vi "I16ArrayToStr(cast).vi"(1 "I16数组":i16[](array[numeric]) format="%.0x") -> (0 "字符串":string)   [LabVIEW 2012]
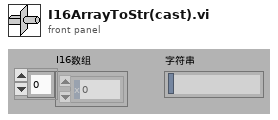
[diagram p1: front panel]
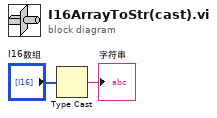
[diagram p0: block diagram]
diagram:
  n1 = Type Cast(x="I16数组") -> (*(type *) &x=→"字符串":string)  [unwired: 1 in]
